vi "Find Shared Variable from URL.vi"(10 "Target List":string[](array[string]), 11 "Variable List":refnum<class "ChannelVS.lvclass">[](array[class])) -> (2 "Sort Name List":string[](array[string]), 3 "Variable info":refnum<class "ChannelVS.lvclass">[](array[class]))   [LabVIEW 2020, in "Shared Variables CD 2.0 Configuration.lvlib" / "ChannelVS.lvclass"]
uses:
  ChannelVS.lvclass
  Public/Documents/National Instruments/NI VeriStand 2020/Custom Devices/Shared Variables CD 2.0/Data/Channel.lvlibp/Channel.lvclass
  C:/Users/Public/Documents/National Instruments/NI VeriStand 2020/Custom Devices/Shared Variables CD 2.0/Data/Channel.lvlibp/Channel.lvclass
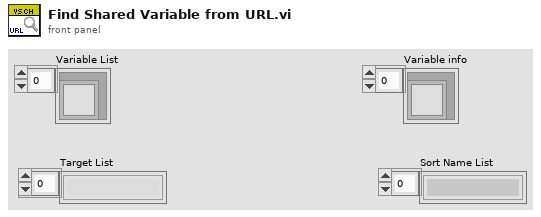
[diagram p1: front panel]
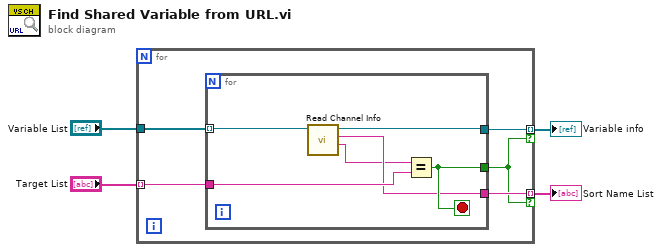
[diagram p0: block diagram]
diagram:
  n1 = for {
    tunnel: "Target List" -> [w9] mode=indexing
    tunnel: "Variable List" -> [w8]
    tunnel: [w7] -> w1 mode=indexing if=w5
    tunnel: [w6] -> w2 mode=indexing if=w5
    n2 = for {
      tunnel: w9 -> [w15]
      tunnel: w8 -> [w11] mode=indexing
      tunnel: [w10] -> w7
      tunnel: [w14] -> w5
      tunnel: [w13] -> w6
      stop <- w14 stop-if-true
      n3 = call "Read Channel Info.vi"("Channel in"=w11) -> ("URL"=w12:string, "Name"=w13:string, "Channel out"=w10:refnum<class "ChannelVS.lvclass">)  [unwired: 5 in, 3 out]
      n4 = Equal?(x=w12, y=w15) -> (x = y?=w14:bool)
    }
  }
  "Variable info" <- w1
  "Sort Name List" <- w2
